vi "example2.vi"() -> ()   [LabVIEW 2015]
panel:
  out "Numeric \nIndicator":dbl
  in  "Numeric\nControl":dbl
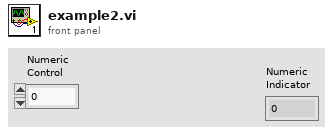
[diagram p1: front panel]
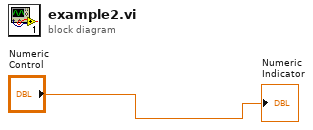
[diagram p0: block diagram]
diagram:
  "Numeric \nIndicator" <- "Numeric\nControl"
